vi "Motor Encoder Global.vi"() -> ()   [LabVIEW 2009]
panel:
  in  "stop":bool
  out "Lidar Encoder Index":bool
  out "Steering Encoder Index":bool
  out "Drive Encoder Index":bool
  out "Lidar Encoder B":bool
  out "Steering Encoder B":bool
  out "Drive Encoder B":bool
  out "Lidar Encoder A":bool
  out "Steering Encoder A":bool
  out "Drive Encoder A":bool
  in  "Lidar Encoder":i32
  in  "Steering Encoder":i32
  in  "Drive Encoder":i32
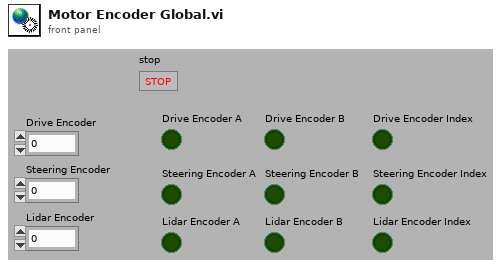
[diagram p1: front panel]
diagram:
